vi "Instance.vi"(8 "error in (no error)":errorcluster) -> (0 "error out":errorcluster, 3 "App out":refnum<class "App.lvclass">)   [LabVIEW 2020, in "PicoG-App.lvlib" / "App.lvclass"]
uses:
  App.lvclass
  <vilib>/ErrorRing/Error Ring.xnode
  <vilib>/Utility/error.llb/Error Cluster From Error Code.vi
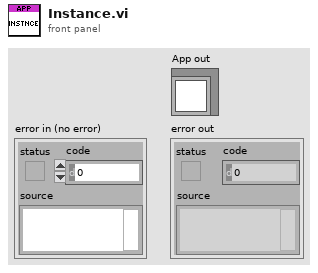
[diagram p1: front panel]
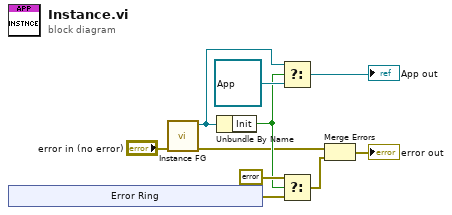
[diagram p0: block diagram]
diagram:
  n1 = xnode "Error Ring"() -> ("error out"=w6:errorcluster)
  n2 = call "Instance FG.vi"("error in (no error)"="error in (no error)") -> ("error out"=w3:errorcluster, "App out"=w9:refnum<class "App.lvclass">)  [unwired: 9 in]
  n3 = Unbundle By Name(w9) -> ("Init"=w4:bool)
  n4 = Select(t=w9, s=w4, f=refnum<class "App.lvclass"> refnum ("App out")) -> (s? t:f=→"App out":refnum<class "App.lvclass">)
  n5 = Select(t=errorcluster {"status"=FALSE, "code"=0, "source"=""}, s=w4, f=w6) -> (s? t:f=w2:errorcluster)
  n6 = Merge Errors(w3, w2) -> (→"error out":errorcluster)
